vi "Main.vi"() -> ()   [LabVIEW 2017]
uses:
  <extravilib>/ChannelInstances/Messenger-bool/Write With Abort.vi
  <resource>/Channels/Messenger/Write With Abort.vi
  <extravilib>/ChannelInstances/Messenger-bool/Wrapper.lvclass
  C:/Program Files (x86)/National Instruments/LabVIEW 2017/vi.lib/ChannelSupport/Channel Message/Channel Message.lvclass
  <extravilib>/ChannelInstances/Messenger-bool/Instantiate.vi
  <extravilib>/ChannelInstances/Messenger-bool/Wrap.vi
  <resource>/Channels/Messenger/Endpoint.vi
  <extravilib>/ChannelInstances/Messenger-bool.lvlib
panel:
  out "Quit?":bool
  in  "Start":bool
  in  "Exit":bool
  out "Last Measurement":dbl
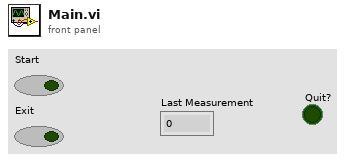
[diagram p1: front panel]
types:
  T1 = typedef "Messenger-bool.lvlib/))Channel.ctl" = refnum<queue>
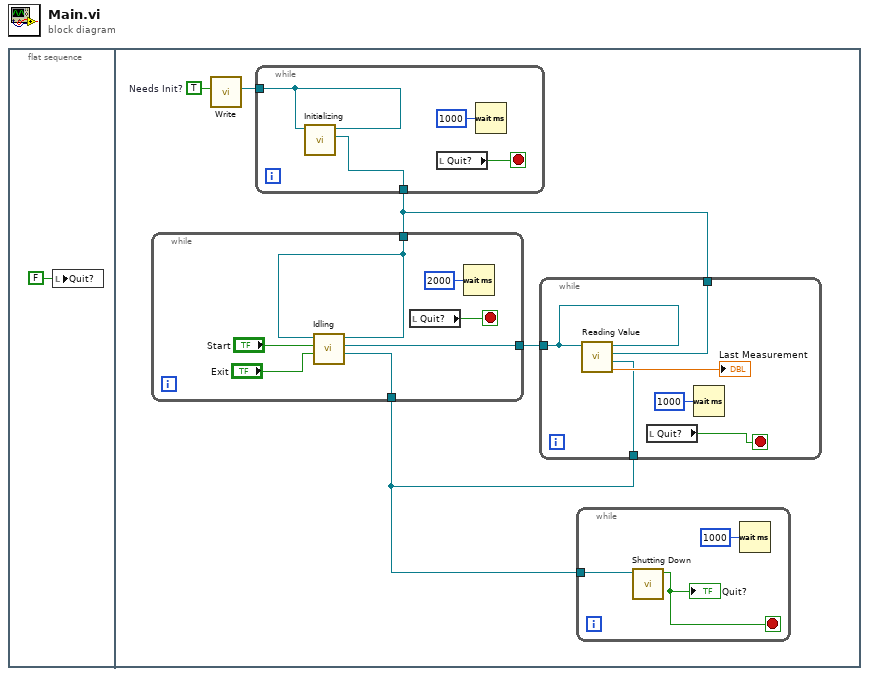
[diagram p0: block diagram]
diagram:
  n1 = flat-sequence {
    frame #0 {
      n2 = local write "Quit?"(FALSE ("Quit?")) -> ()
    }
    frame #1 {
      w6 = TRUE  # Needs Init?
      n3 = while {
        tunnel: [w23] -> w5
        tunnel: [w21] -> w4
        tunnel: [w20] -> w2
        stop <- w22 stop-if-true
        n4 = call "Idling.vi"("Exit"="Exit", "Start"="Start", "Go to Idle?"=w21) -> ("Exit"=w20:T1, "Make Measurement"=w23:T1, "Return to Idling"=w21:T1)  [unwired: 6 in]
        n5 = local read "Quit?"() -> (w22:bool)
        n6 = Wait (ms)(milliseconds to wait=u32 2000) -> ()  [unwired: 1 out]
      }
      n7 = call <extravilib>:"Write.vi"("element"=w6) -> ("channel"=w3:T1)  [unwired: 8 in, 2 out]
      n8 = while {
        tunnel: w4 -> [w8]
        tunnel: w3 -> [w7]
        stop <- w10 stop-if-true
        n9 = call "Initializing.vi"("Retry Initialization"=w7, "Needs Init?"=w7) -> ("Go to Idling"=w8:T1)  [unwired: 9 in]
        n10 = local read "Quit?"() -> (w10:bool)
        n11 = Wait (ms)(milliseconds to wait=u32 1000) -> ()  [unwired: 1 out]
      }
      n12 = while {
        tunnel: w5 -> [w15]
        tunnel: w4 -> [w14]
        tunnel: w2 -> [w13]
        stop <- w11 stop-if-true
        n13 = call "Reading Value.vi"(3:"Measure"=w15, 11:"Measure"=w15) -> ("Last Measurement"=→"Last Measurement":dbl, "Exit!"=w13:T1, "Go to Idle"=w14:T1)  [unwired: 7 in]
        n14 = local read "Quit?"() -> (w11:bool)
        n15 = Wait (ms)(milliseconds to wait=u32 1000) -> ()  [unwired: 1 out]
      }
      n16 = while {
        tunnel: w2 -> [w18]
        stop <- w19 stop-if-true
        n17 = call "Shutting Down.vi"("Exit"=w18) -> ("Quit?"=w19:bool)  [unwired: 10 in]
        "Quit?" <- w19
        n18 = Wait (ms)(milliseconds to wait=u32 1000) -> ()  [unwired: 1 out]
      }
    }
  }
